vi "API String to 1D Array 2.vi"(4 "SEPERATOR":enum16{"0x2C - ,", "0x3B - ;"}(ring), 8 "Error in":errorcluster caption="Error in (no error)", 10 "string":string) -> (0 "Error out":errorcluster, 2 "Array of Strings":string[](array[string])=["sin(x)+2", "VIA(x", "y)", " VIB(z)"])   [LabVIEW 2017]
uses:
  <userlib>/_NEVSTOP/Communicable State Machine(CSM)/Communicable State Machine.lvlib
  API-String-Arugments-Support/API String Arguments Support.lvlib
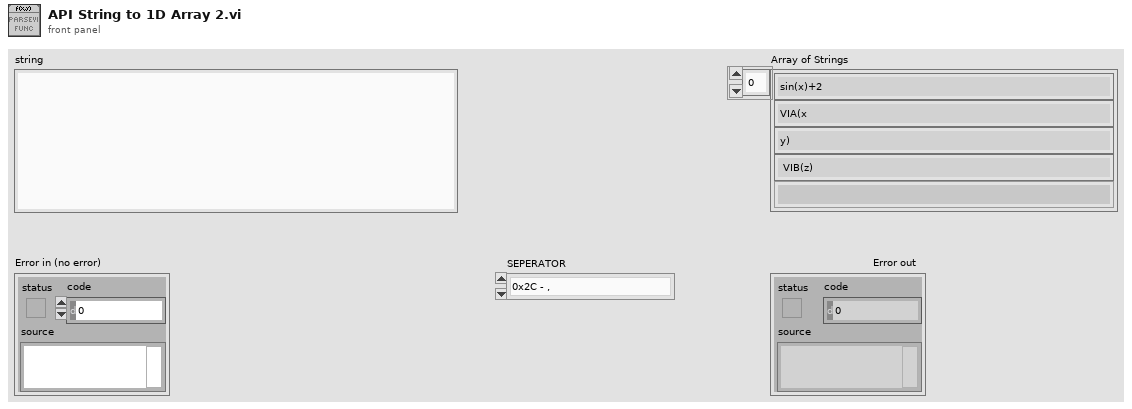
[diagram p1: front panel]
types:
  T1 = enum16{"0x2829 - ()", "0x5B5D - []", "0x7B7D - {}"}
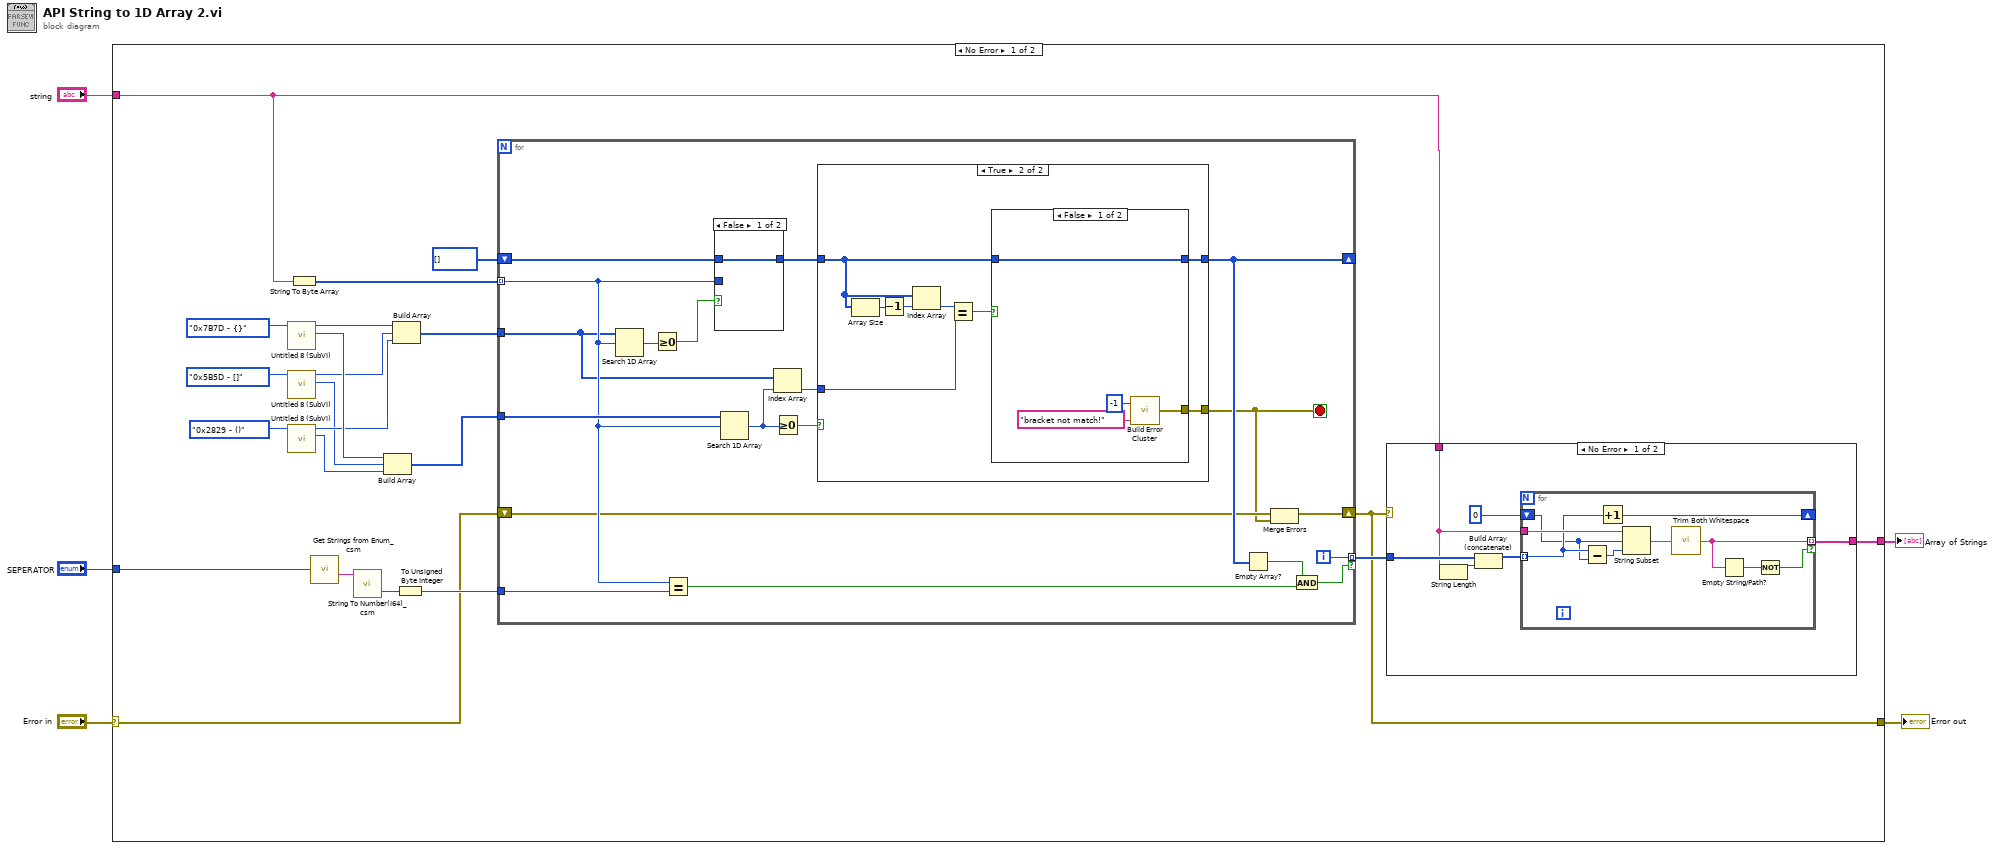
[diagram p0: block diagram]
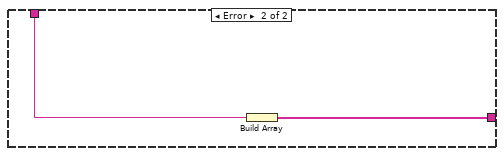
[diagram p2: hidden frame]
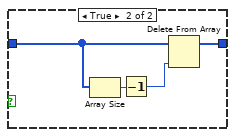
[diagram p4: hidden frame]
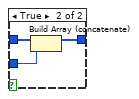
[diagram p5: hidden frame]
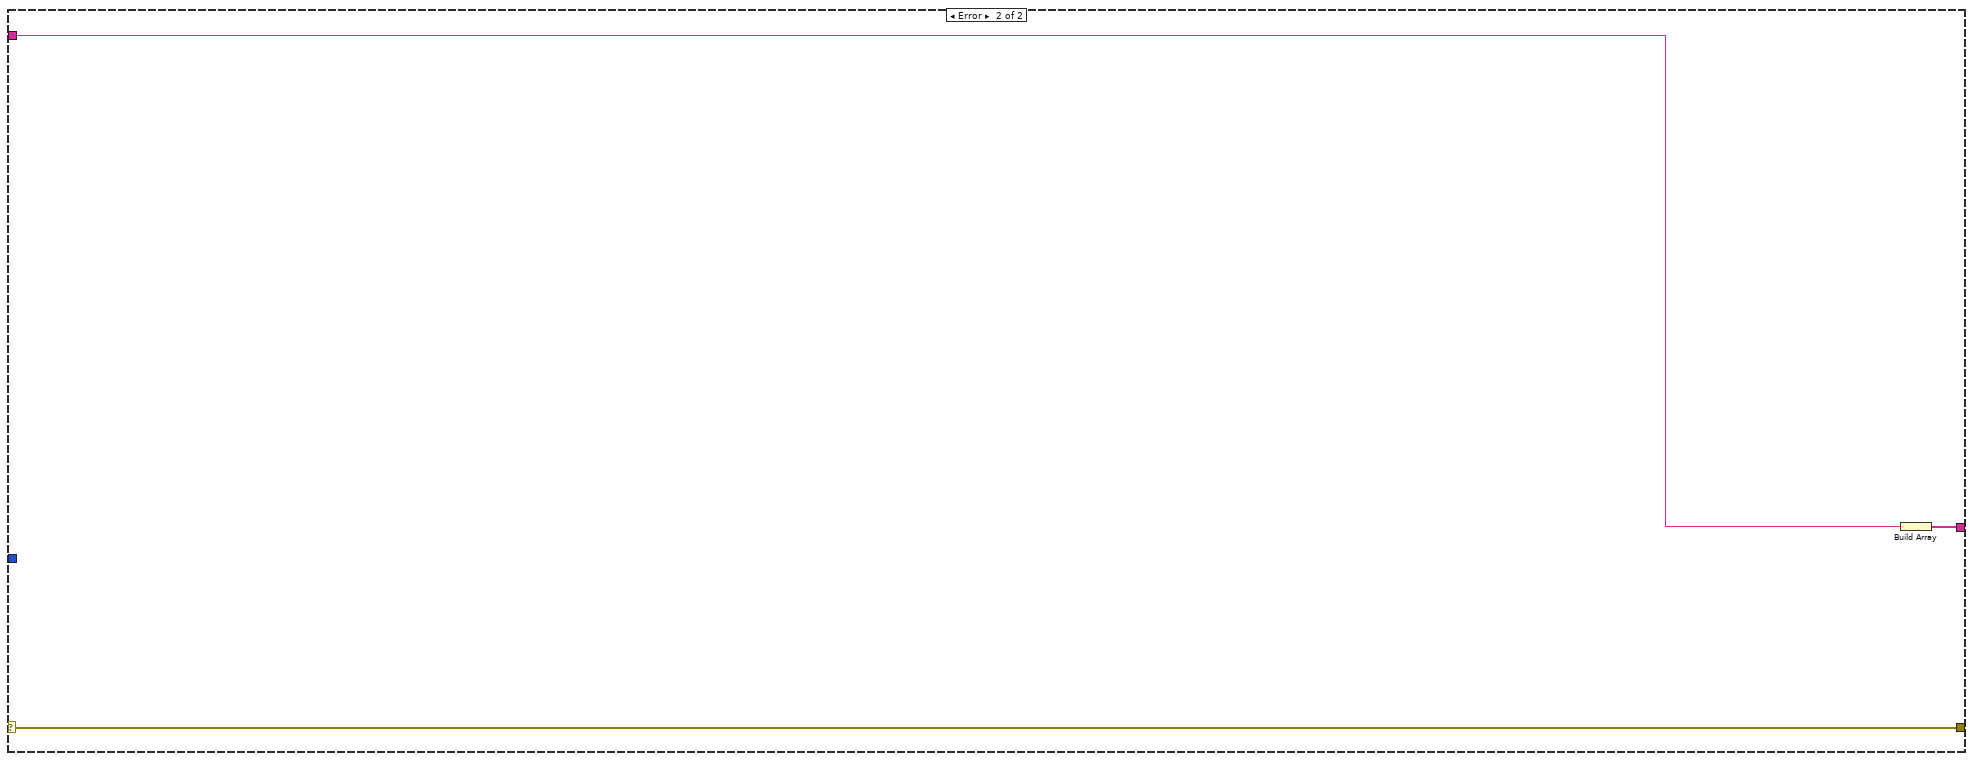
[diagram p6: hidden frame]
diagram:
  n1 = case shown="No Error" "Error in" {
    selector: "Error in" -> [w8 w87]
    tunnel: [w24 w86] -> w5
    tunnel: "string" -> [w18 w85]
    tunnel: [w7 w87] -> w2
    tunnel: "SEPERATOR" -> [w6 _]
    frame No Error {
      n2 = call "Untitled 8 (SubVI).vi"("Enum"=T1."0x7B7D - {}" ("TYPE")) -> ("Numeric"=w14:u8, "Numeric 2"=w22:u8)  [unwired: 9 in]
      n3 = call "Untitled 8 (SubVI).vi"("Enum"=T1."0x5B5D - []" ("TYPE")) -> ("Numeric"=w11:u8, "Numeric 2"=w13:u8)  [unwired: 9 in]
      n4 = call "Untitled 8 (SubVI).vi"("Enum"=T1."0x2829 - ()" ("TYPE")) -> ("Numeric"=w10:u8, "Numeric 2"=w12:u8)  [unwired: 9 in]
      n5 = String To Byte Array(string=w18) -> (unsigned byte array=w26:u8[])
      n6 = call <userlib>:"Get Strings from Enum_csm.vi"("Enum"=w6) -> ("String Value"=w21:string)  [unwired: 7 in, 3 out]
      n7 = call "String To Number(I64)_csm.vi"("String"=w21) -> ("Numeric(I64)"=w20:u64)  [unwired: 4 in]
      n8 = Build Array(w14, w11, w10) -> (w9:u8[])
      n9 = Build Array(w22, w13, w12) -> (w15:u8[])
      n10 = To Unsigned Byte Integer(number=w20) -> (unsigned 8bit integer=w19:u8)
      n11 = for {
        tunnel: w26 -> [w51] mode=indexing
        shift-right: [w59] -> _
        shift-left: u8[] [] -> [w62]
        tunnel: [w61] -> w25 mode=indexing if=w58
        tunnel: w15 -> [w46]
        tunnel: w9 -> [w53]
        tunnel: w19 -> [w56]
        shift-right: [w49] -> w7
        shift-left: w8 -> [w50]
        i -> [w61]
        stop <- w48 stop-if-true
        n12 = Search 1D Array(1D array=w46, element=w51) -> (index of element=w55:i32)  [unwired: 1 in]
        n13 = Greater Or Equal To 0?(x=w55) -> (x >= 0?=w54:bool)
        n14 = Equal?(x=w51, y=w56) -> (x = y?=w57:bool)
        n15 = case shown="False" w54 {
          tunnel: w62 -> [w81 w84]
          tunnel: w51 -> [_ w83]
          tunnel: [w81 w82] -> w63
          frame False {
          }
          frame True {
            n16 = Build Array (concatenate)(w84, w83) -> (w82:u8[])
          }
        }
        n17 = Search 1D Array(1D array=w53, element=w51) -> (index of element=w45:i32)  [unwired: 1 in]
        n18 = Index Array(array=w46, index=w45) -> (element=w47:u8)
        n19 = Greater Or Equal To 0?(x=w45) -> (x >= 0?=w52:bool)
        n20 = case shown="True" w52 {
          tunnel: w63 -> [w64 w69]
          tunnel: [w64 w72] -> w59
          tunnel: w47 -> [_ w67]
          tunnel: [_ w65] -> w48
          frame False {
          }
          frame True {
            n21 = Array Size(array=w69) -> (size(s)=w71:i32)
            n22 = Decrement(x=w71) -> (x-1=w70:i32)
            n23 = Index Array(array=w69, index=w70) -> (element=w68:u8)
            n24 = Equal?(x=w68, y=w67) -> (x = y?=w66:bool)
            n25 = case shown="False" w66 {
              tunnel: w69 -> [w76 w79]
              tunnel: [w76 w77] -> w72
              tunnel: [w73 _] -> w65
              frame False {
                n26 = call <userlib>:"Build Error Cluster.vi"("String to Prepend to source (\"\")"="bracket not match!" ("String to Prepend to source (\"\")"), "code"=-1) -> ("error out"=w73:errorcluster)
              }
              frame True {
                n27 = Array Size(array=w79) -> (size(s)=w80:i32)
                n28 = Decrement(x=w80) -> (x-1=w78:i32)
                n29 = Delete From Array(array=w79, index=w78) -> (array with subset deleted=w77:u8[])  [unwired: 1 in, 1 out]
              }
            }
          }
        }
        n30 = Empty Array?(array=w59) -> (empty?=w60:bool)
        n31 = Merge Errors(w50, w48) -> (w49:errorcluster)
        n32 = And(x=w60, y=w57) -> (x .and. y?=w58:bool)
      }
      n33 = case shown="No Error" w7 {
        tunnel: w25 -> [w33 _]
        tunnel: [w31 w43] -> w24
        tunnel: w18 -> [w28 w44]
        frame No Error {
          n34 = String Length(string=w28) -> (length=w29:i32)
          n35 = Build Array (concatenate)(w33, w29) -> (w30:i32[])
          n36 = for {
            tunnel: w28 -> [w42]
            tunnel: w30 -> [w40] mode=indexing
            tunnel: [w36] -> w31 mode=indexing if=w34
            shift-right: [w37] -> _
            shift-left: 0 ("Numeric") -> [w38]
            n37 = Subtract(x=w40, y=w38) -> (x-y=w39:i32)
            n38 = Increment(x=w40) -> (x+1=w37:i32)
            n39 = String Subset(string=w42, offset (0)=w38, length (rest)=w39) -> (substring=w41:string)
            n40 = call <userlib>:"Trim Both Whitespace.vi"("string"=w41) -> ("trimmed string"=w36:string)  [unwired: 1 in]
            n41 = Empty String/Path?(string/path=w36) -> (empty?=w35:bool)
            n42 = Not(x=w35) -> (.not. x?=w34:bool)
          }
        }
        frame Error {
          n43 = Build Array(w44) -> (w43:string[])
        }
      }
    }
    frame Error {
      n44 = Build Array(w85) -> (w86:string[])
    }
  }
  "Array of Strings" <- w5
  "Error out" <- w2
